vi "Validate Rate (No Objects).vi"(8 "error IO":errorcluster, 10 "rate":dbl[unit] caption="Rate", 11 "Cluster In":T4={"Field"=0.0, "Rate"=0.0, "Status"={"Sweeping"=FALSE, "Clamped"=FALSE, "Hold"=FALSE, "At Rest"=FALSE, "Quench"=FALSE, "Persistent Mode"=FALSE, "Switch Heater"=FALSE}, "ILM Shut Down?"=FALSE, "IO Info"={"Address"={"Com Port"=1, "ISOBUS Address"=2, "GPIB Address"=24, "Communication"=enum."ISOBUS"}, "Version"=enum."IPS"}, "IO Info (Level Meter)"={"Address"={"Com Port"=1, "ISOBUS Address"=5, "GPIB Address"=24, "Communication"=enum."ISOBUS"}, "ILM Name"="", "Display Channel"=[]}, "Training?"=FALSE, "Training Field and Speed Cluster"={"Training Field"=[0.0, 4.108, 5.78, 8.001], "Training Speed"=[0.0057, 0.0022833333333333334, 0.0011333333333333334, 0.0011333333333333334]}}) -> (0 "error out":errorcluster, 1 "Max rate":dbl[unit], 2 "Coerced rate":dbl[unit], 3 "Cluster Out":T4={"Field"=0.0, "Rate"=0.0, "Status"={"Sweeping"=FALSE, "Clamped"=FALSE, "Hold"=FALSE, "At Rest"=FALSE, "Quench"=FALSE, "Persistent Mode"=FALSE, "Switch Heater"=FALSE}, "ILM Shut Down?"=FALSE, "IO Info"={"Address"={"Com Port"=1, "ISOBUS Address"=2, "GPIB Address"=24, "Communication"=enum."ISOBUS"}, "Version"=enum."IPS"}, "IO Info (Level Meter)"={"Address"={"Com Port"=1, "ISOBUS Address"=5, "GPIB Address"=24, "Communication"=enum."ISOBUS"}, "ILM Name"="", "Display Channel"=[]}, "Training?"=FALSE, "Training Field and Speed Cluster"={"Training Field"=[0.0, 4.108, 5.78, 8.001], "Training Speed"=[0.0057, 0.0022833333333333334, 0.0011333333333333334, 0.0011333333333333334]}}, 4 "Coerced?":bool, 6 "Field":dbl[unit])   [LabVIEW 2009]
doc: "Query the current field and verify that the given sweep rate is appropriate for this field."
uses:
  Magnet status.ctl
  Oxford/PSSUBS.LLB/PSIO.ctl
  Oxford/BUSGEN.LLB/OxfordAddress.ctl
  Power Supply.lvclass
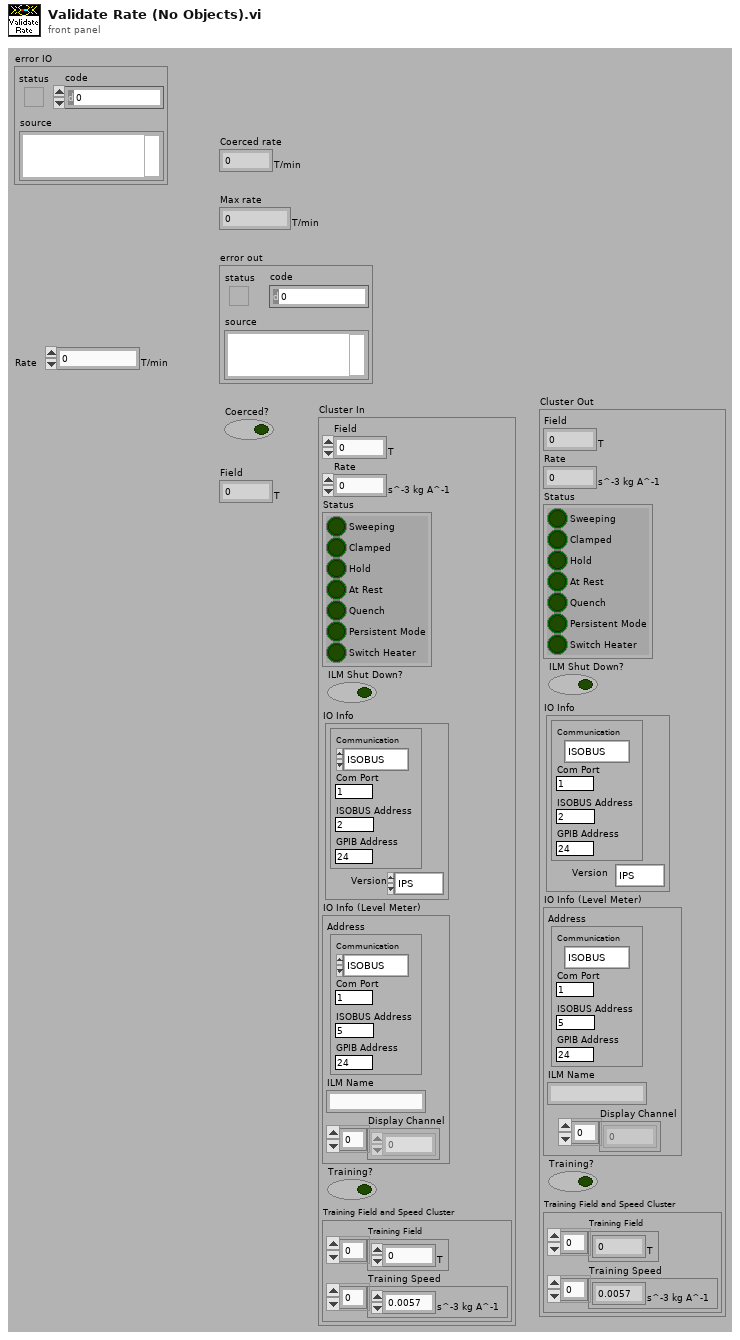
[diagram p1: front panel]
types:
  T1 = typedef "Power Supply.lvclass/Magnet status.ctl" = cluster{"Sweeping":bool, "Clamped":bool, "Hold":bool, "At Rest":bool, "Quench":bool, "Persistent Mode":bool, "Switch Heater":bool}
  T2 = typedef "PSIO.ctl" = cluster{"Address":T3, "Version":enum16{"PS", "IPS"}}
  T3 = typedef "OxfordAddress.ctl" = cluster{"Com Port":i32, "ISOBUS Address":i32, "GPIB Address":i16, "Communication":enum16{"RS232", "ISOBUS", "GPIB", "Gateway"}}
  T4 = cluster{"Field":dbl[unit], "Rate":dbl[unit], "Status":T1, "ILM Shut Down?":bool, "IO Info":T2, "IO Info (Level Meter)":cluster{"Address":T3, "ILM Name":string, "Display Channel":i32[]}, "Training?":bool, "Training Field and Speed Cluster":cluster{"Training Field":dbl[unit][], "Training Speed":dbl[unit][]}}
  T5 = cluster{"Training Field":dbl[unit][], "Training Speed":dbl[unit][]}
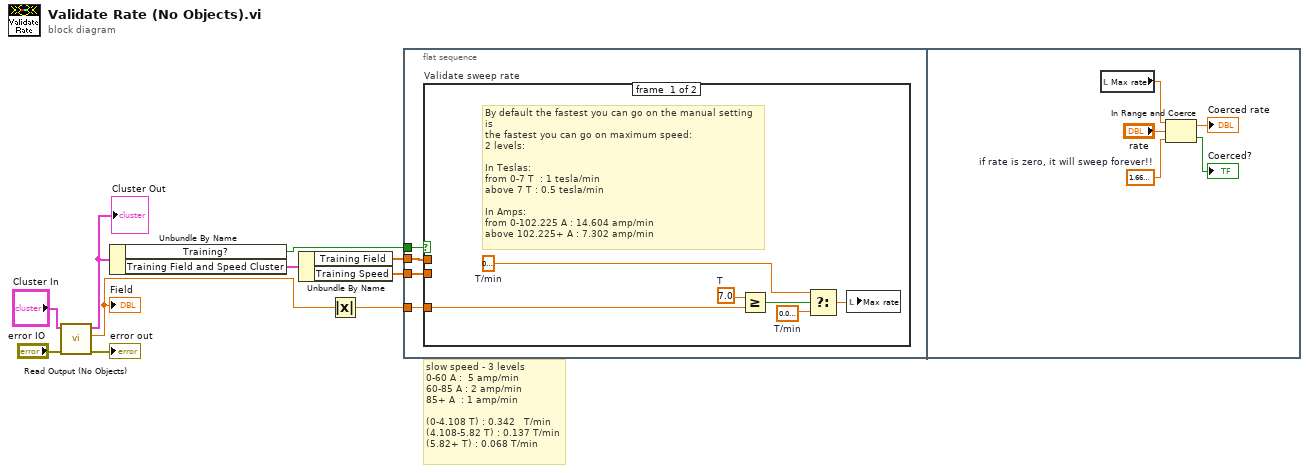
[diagram p0: block diagram]
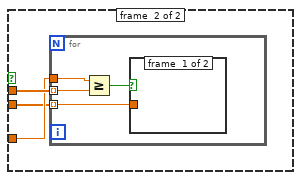
[diagram p2: hidden frame]
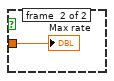
[diagram p3: hidden frame]
diagram:
  # "slow speed - 3 levels\n0-60 A :  5 amp/min\n60-85 A : 2 amp/min\n85+ A  : 1 amp/min\n\n(0-4.108 T) : 0.342   T/min\n(4.108-5.82 T) : 0.137 T/min\n(5.82+ T) : 0.068 T/min"
  n1 = call "Read Output (No Objects).vi"("error in (no error)"="error IO", "Cluster In"="Cluster In") -> ("error out"=→"error out":errorcluster, "Field"=w10:dbl[unit], "Cluster Out"=w1:T4)  [unwired: 6 in, 1 out]
  "Field" <- w10
  "Cluster Out" <- w1
  n2 = Unbundle By Name(w1) -> ("Training?"=w6:bool, "Training Field and Speed Cluster"=w5:T5)
  n3 = Unbundle By Name(w5) -> ("Training Field"=w4:dbl[unit][], "Training Speed"=w3:dbl[unit][])
  n4 = Absolute Value(x=w10) -> (abs(x)=w7:dbl[unit])
  n5 = flat-sequence {
    tunnel: w7 -> [w14]
    tunnel: w6 -> [w13]
    tunnel: w4 -> [w12]
    tunnel: w3 -> [w11]
    frame #0 {
      n6 = case "Validate sweep rate" shown="True" w13 {
        tunnel: w14 -> [w16 w22]
        tunnel: w12 -> [_ w23]
        tunnel: w11 -> [_ w21]
        frame #0 {
          w18 = dbl[unit] 0.008333333333333333  # T/min
          w17 = dbl[unit] 0.016666666666666666  # T/min
          w19 = dbl[unit] 7.0  # T
          # "By default the fastest you can go on the manual setting is\nthe fastest you can go on maximum speed:\n2 levels:\n\nIn Teslas:\nfrom 0-7 T  : 1 tesla/min\nabove 7 T : 0.5 tesla/min\n\nIn Amps:\nfrom 0-102.225 A : 14.604 amp/min\nabove 102.225+ A : 7.302 amp/min"
          n7 = Greater Or Equal?(x=w19, y=w16) -> (x >= y?=w20:bool)
          n8 = Select(t=w17, s=w20, f=w18) -> (s? t:f=w15:dbl[unit])
          n9 = local write "Max rate"(w15) -> ()
        }
        frame #1 {
          n10 = for {
            tunnel: w23 -> [w27] mode=indexing
            tunnel: w22 -> [w26]
            tunnel: w21 -> [w24] mode=indexing
            n11 = Greater Or Equal?(x=w26, y=w27) -> (x >= y?=w25:bool)
            n12 = case shown="True" w25 {
              tunnel: w24 -> [_ w28]
              frame #0 {
              }
              frame #1 {
                "Max rate" <- w28
              }
            }
          }
        }
      }
    }
    frame #1 {
      w29 = dbl[unit] 1.6666666666666667e-08  # if rate is zero, it will sweep forever!!
      n13 = local read "Max rate"() -> (w33:dbl[unit])
      n14 = In Range and Coerce(upper limit=w33, x="rate", lower limit=w29) -> (coerced(x)=→"Coerced rate":dbl[unit], In Range?=→"Coerced?":bool)
    }
  }
